vi "Create Logger.vi"(7 "framework options":T1={"FIFO Options"={"Infinite Timeouts"=FALSE}, "Thread Options"={"Show FP On Call"=FALSE, "Close FP After Call"=FALSE, "Allow Debugging"=FALSE}, "Plugin Options"={"Default Components"=FALSE}, "Performance Options"={"Measure Period"=FALSE, "Measure Rx/Tx Duration"=FALSE}, "Data Server Options"={"Enable Data Server"=FALSE, "Period"=50}} {"Data Server Options"."Period" format="%d ms"}, 8 "error in (no error)":errorcluster, 10 "log file directory":path, 11 "Framework in":refnum<class "Framework.lvclass">) -> (0 "error out":errorcluster, 1 "Logging Interface":refnum<class "Logging Interface.lvclass">, 2 "Logging Thread":refnum<class "Logging Thread.lvclass">, 3 "Framework out":refnum<class "Framework.lvclass">)   [LabVIEW 2019, in "DSF Core.lvlib" / "Framework.lvclass"]
uses:
  Framework.lvclass
  Thread/Logging/Logging Thread.lvclass
  C:/Dev/GitHub/niveristand-data-sharing-framework-custom-device/Core/Classes/Thread/Thread.lvclass
  Framework Options.ctl
  Typedefs/DSF FIFO Options.ctl
  Thread/Thread Options.ctl
  Typedefs/DSF Plugin Options.ctl
  Typedefs/DSF Performance Options.ctl
  Data Server Options.ctl
  Interface/Logging/Logging Interface.lvclass
  C:/Dev/GitHub/niveristand-data-sharing-framework-custom-device/Core/Classes/Interface/Interface.lvclass
  Thread/Thread Settings.ctl
  Thread/Thread.lvclass/Thread.ctl
  Interface/Interface.lvclass/Interface.ctl
  Thread/Logging/Logging Thread.lvclass/Logging Thread.ctl
  Framework.lvclass/Framework.ctl
  Interface/Logging/Create.vi
  Thread/Set Name.vi
  Thread/Set Thread Parameters.vi
  Thread/Logging/Create Log File.vi
  Interface/New Interface.vi
  Interface/Create RT FIFO.vi
  Thread/Thread.lvclass
  DSF Core.lvlib
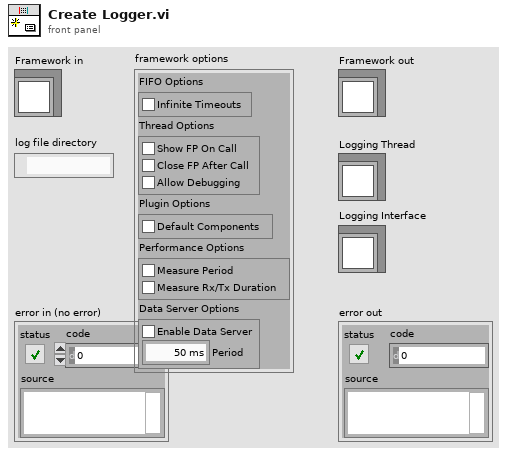
[diagram p1: front panel]
types:
  T1 = typedef "DSF Core.lvlib/Framework.lvclass/Framework Options.ctl" = cluster{"FIFO Options":T2, "Thread Options":T3, "Plugin Options":T4, "Performance Options":T5, "Data Server Options":T6}
  T2 = typedef "DSF Core.lvlib/Framework.lvclass/DSF FIFO Options.ctl" = cluster{"Infinite Timeouts":bool}
  T3 = typedef "DSF Core.lvlib/Thread.lvclass/Thread Options.ctl" = cluster{"Show FP On Call":bool, "Close FP After Call":bool, "Allow Debugging":bool}
  T4 = typedef "DSF Core.lvlib/Framework.lvclass/DSF Plugin Options.ctl" = cluster{"Default Components":bool}
  T5 = typedef "DSF Core.lvlib/DSF Performance Options.ctl" = cluster{"Measure Period":bool, "Measure Rx/Tx Duration":bool}
  T6 = typedef "DSF Core.lvlib/Framework.lvclass/Data Server Options.ctl" = cluster{"Enable Data Server":bool, "Period":u32}
  T7 = typedef "DSF Core.lvlib/Thread.lvclass/Thread Settings.ctl" = cluster{"Priority":u16, "Processor":i32}
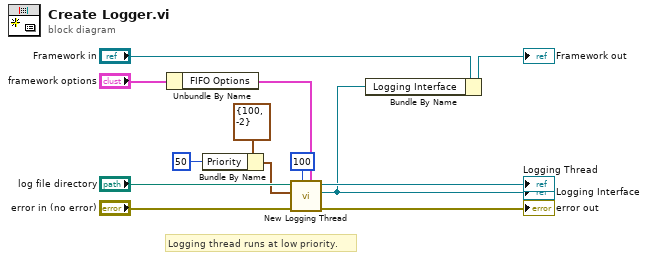
[diagram p0: block diagram]
diagram:
  # "Logging thread runs at low priority."
  n1 = Unbundle By Name("framework options") -> ("FIFO Options"=w5:T2)
  n2 = Bundle By Name(cluster=T7 {"Priority"=100, "Processor"=-2} ("Thread Parameters"), "Priority"=u16 50 ("priority (100)")) -> (w1:T7)
  n3 = call "New Logging Thread.vi"("FIFO Options"=w5, "fifo depths (100)"=u32 100 ("fifo depths"), "error in (no error)"="error in (no error)", "thread settings"=w1, "log file directory"="log file directory") -> ("error out"=→"error out":errorcluster, "Logging Interface"=w3:refnum<class "Logging Interface.lvclass">, "Logging Thread out"=→"Logging Thread":refnum<class "Logging Thread.lvclass">)  [unwired: 4 in]
  "Logging Interface" <- w3
  n4 = Bundle By Name(cluster="Framework in", "Logging Interface"=w3) -> (→"Framework out":refnum<class "Framework.lvclass">)
